vi "Test Executive to Data Type.vi"(8 "error in (no error)":errorcluster, 11 "Test Executive Ref":refnum<data-value>) -> (0 "error out":errorcluster, 3 "Boolean out":refnum<class "Test Executive.lvclass">)   [LabVIEW 2017, in "Custom Type Test Executive.lvlib" / "Test Executive.lvclass"]
uses:
  <vilib>/gpm_packages/@cs/test-executive/Source/Custom Type Test Executive/Test Executive Data Type/Test Executive.lvclass
  <vilib>/gpm_packages/@cs/test-executive/Source/Test Executive/ITestExecutive/ITest Executive.lvclass
  <vilib>/gpm_packages/@cs/test-executive/Source/Custom Type Test Executive/Test Executive Data Type/Test Executive.lvclass/Test Executive.ctl
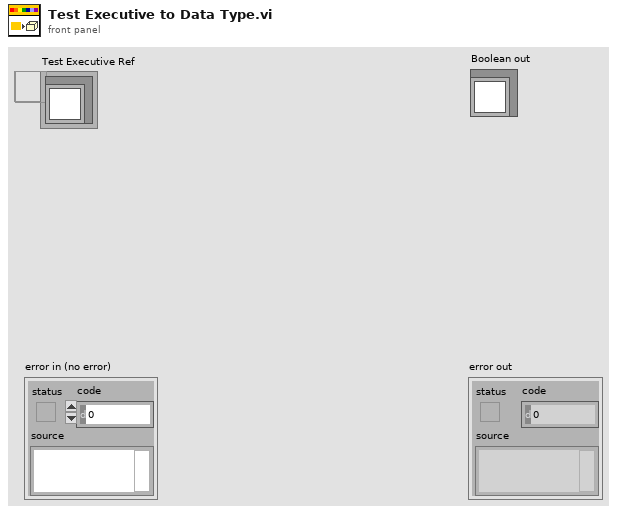
[diagram p1: front panel]
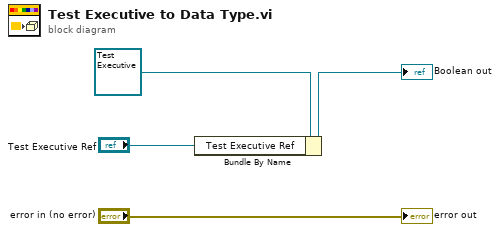
[diagram p0: block diagram]
diagram:
  n1 = Bundle By Name(cluster=refnum<class "Test Executive.lvclass"> refnum ("Boolean in"), "Test Executive Ref"="Test Executive Ref") -> (→"Boolean out":refnum<class "Test Executive.lvclass">)
  "error out" <- "error in (no error)"
